vi "Compose LabVIEW Object - Aggregate - Value.vi"() -> ()   [LabVIEW 2017, in "Composition.Tests.lvlib"]
uses:
  Composition.Tests.lvlib
  c53c5236-6a32-4dca-880e-4ad1106e00ac.vi
  Classes/Aggregate/Aggregate.lvclass
  Classes/String/String.lvclass
  Classes/Child/Child.lvclass
  <vilib>/addons/_JKI Toolkits/Caraya/classes/Assert/Assert.lvclass
  <vilib>/addons/_JKI Toolkits/Caraya/classes/Test/Test.lvclass
panel:
  out "error out":errorcluster
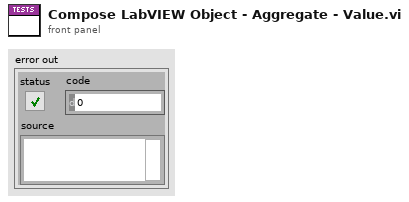
[diagram p1: front panel]
types:
  T1 = cluster{"Major":u16, "Minor":u16, "Fix":u16, "Build":u16}[]
  T2 = cluster{"String out":refnum<class "String.lvclass">, "Child out":refnum<class "Child.lvclass">}
  T3 = cluster{"String out":refnum<class "String.lvclass">, "Child out":refnum<class "Child.lvclass">}[]
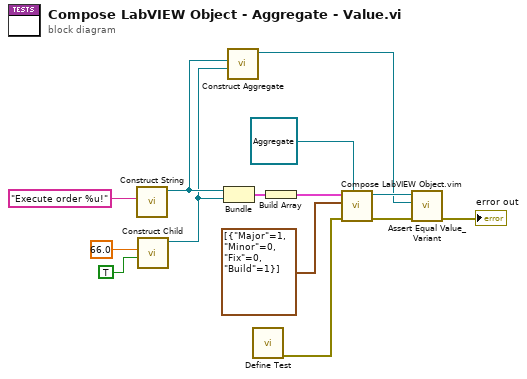
[diagram p0: block diagram]
diagram:
  n1 = call "Construct String.vi"("String"="Execute order %u!") -> ("String out"=w11:refnum<class "String.lvclass">)  [unwired: 9 in, 1 out]
  n2 = call "Construct Child.vi"("Ignored"=TRUE, "Offset"=66.0) -> ("Child out"=w10:refnum<class "Child.lvclass">)  [unwired: 8 in, 1 out]
  n3 = Bundle("String out"=w11, "Child out"=w10) -> (w13:T2)  [unwired: 1 in]
  n4 = call "Construct Aggregate.vi"("Reflection.Tests.lvlib:Child.lvclass"=w10, "Reflection.Tests.lvlib:String.lvclass"=w11) -> ("Aggregate out"=w2:refnum<class "Aggregate.lvclass">)  [unwired: 8 in, 1 out]
  n5 = call <vilib>:"Define Test.vi"() -> ("error out"=w1:errorcluster)  [unwired: 11 in]
  n6 = Build Array(w13) -> (w12:T3)
  n7 = call "Compose LabVIEW Object.vim"("Type"=refnum<class "Aggregate.lvclass"> refnum ("Reflection.Tests.lvlib:Aggregate.lvclass"), "error in (no error)"=w1, "Library Versions"=T1 [{"Major"=1, "Minor"=0, "Fix"=0, "Build"=1}], "Private Data Clusters"=w12) -> ("error out"=w9:errorcluster, "LabVIEW Object"=w3:refnum<class "Aggregate.lvclass">)  [unwired: 6 in]
  n8 = call <vilib>:"Assert Equal Value_Variant.vi"("error in (no error)"=w9, "Y"=w2, "X"=w3) -> ("error out"=→"error out":errorcluster)  [unwired: 8 in]
